vi "Add User Defined Message.vi"(8 "error in (no error)":errorcluster, 11 "Node Ptr":u64 format="%.0x") -> (0 "error out":errorcluster)   [LabVIEW 2024, in "Diagnostics Addon System Explorer.lvlib"]
uses:
  Diagnostics Addon System Explorer.lvlib
  Addon Shared/Types/Type.ctl
  Addon Shared/Diagnostics Addon Shared.lvlib
  <vilib>/NI VeriStand/Custom Device Tools/Custom Device Utility Library/Custom Device Utility Library.lvlib
panel:
  in  "Tag":string
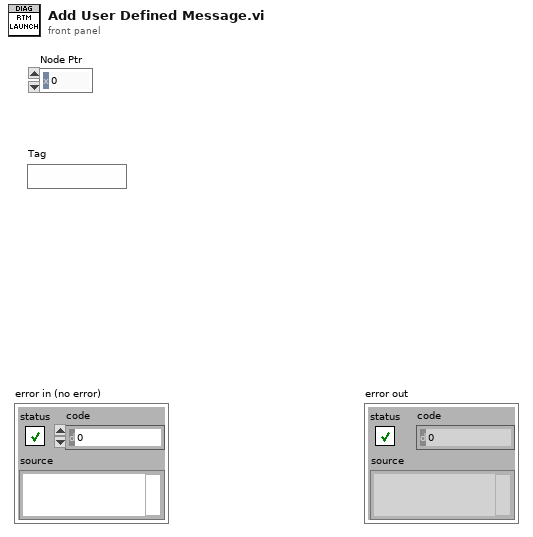
[diagram p1: front panel]
types:
  T1 = typedef "Diagnostics Addon Shared.lvlib/Type.ctl" = enum16{"DID", "CDID", "PID", "CPID", "Read Memory", "Write Memory", "IO Control", "Routine Start", "Routine Request", "Routine Stop", "User Defined", "DTC Control", "Clear DTCs", "Read DTCs", "Start DTCs", "DTC Change Count", "Tester Present", "Unlock ECU", "Reset ECU", "Diag Session Control", "Communication Control", "DPID Control", "Poll Control", "Diag Comm Port Control"}
  T2 = typedef "Custom Device API.lvlib/Custom Device Item Ref.ctl" = u64
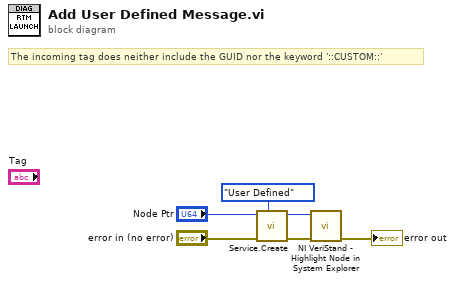
[diagram p0: block diagram]
diagram:
  # "The incoming tag does neither include the GUID nor the keyword '::CUSTOM::'"
  n1 = call "Service.Create.vi"("Type"=Type."User Defined", "error in (no error)"="error in (no error)", "Section Ptr"="Node Ptr") -> ("error out"=w2:errorcluster, "Parent Ref out"=w3:T2)  [unwired: 7 in]
  n2 = call <vilib>:"NI VeriStand - Highlight Node in System Explorer.vi"("error in (no error)"=w2, "Item Ref in"=w3) -> ("error out"=→"error out":errorcluster)  [unwired: 8 in, 1 out]
